vi "Query Status Register.vi"(8 "error in (no error)":errorcluster, 11 "IF_XX in":refnum<class "IF_XX.lvclass">) -> (0 "error out":errorcluster, 3 "IF_XX out":refnum<class "IF_XX.lvclass">)   [LabVIEW 2019, in "IF_XX.lvlib" / "IF_XX.lvclass"]
doc: "The implementation must read status registers and push the status register values to private data for:\nOCP Flag, OVP Flag, Interlock Flag, Output Flag into the private data arrays of the power supply class.\n\nThe routine queries the OVP and OCP registers, Although it is unclear what the return value is expected to be, so we'll have to determine during integration"
uses:
  Library/IF_XX.lvclass
  Library/IF_XX.lvclass/IF_XX.ctl
panel:
  out "Read data 3":string
  out "Read data 2":string
  out "Read data":string
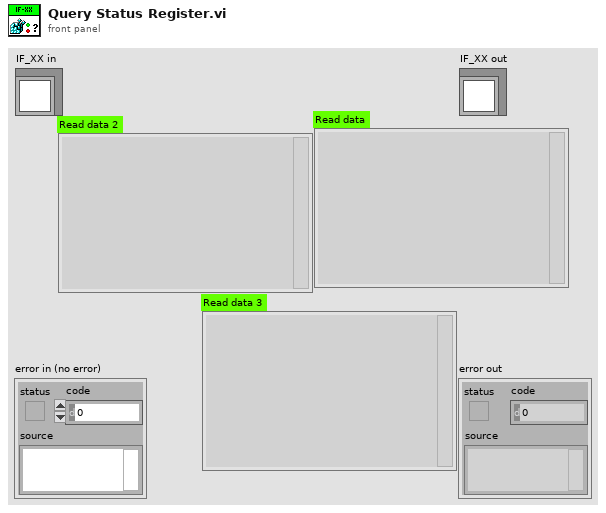
[diagram p1: front panel]
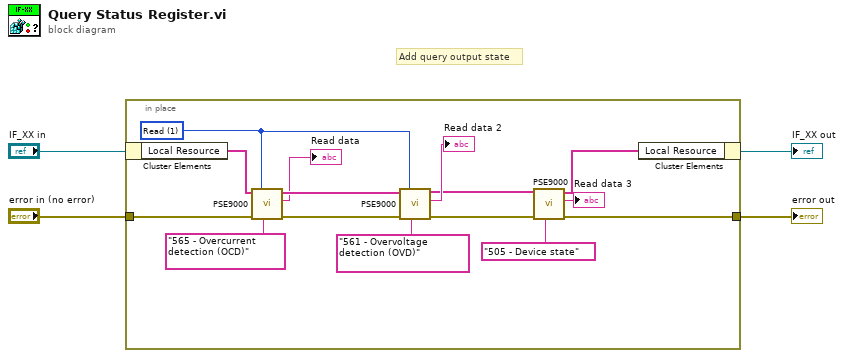
[diagram p0: block diagram]
diagram:
  # "Add query output state"
  n1 = in-place {
    in-place-border: "error in (no error)" -> [w16]
    in-place-border: [w7] -> w1
    w17 = u8 1 items=["Write", "Read"] ("Access")
    n2 = in-place-cluster #1("IF_XX in") -> ("Local Resource"=w18:string[])
    n3 = call <instrlib>:"PSE9000.vi"("Command list"="565 - Overcurrent detection (OCD)", "Error in"=w16, "Access"=w17, "Device information in"=w18) -> ("Error out"=w15:errorcluster, "Read data"=→"Read data":string, "Device information out"=w19:string[])  [unwired: 2 in, 1 out]
    n4 = call <instrlib>:"PSE9000.vi"("Command list"="561 - Overvoltage detection (OVD)", "Error in"=w15, "Access"=w17, "Device information in"=w19) -> ("Error out"=w8:errorcluster, "Read data"=→"Read data 2":string, "Device information out"=w10:string[])  [unwired: 2 in, 1 out]
    n5 = call <instrlib>:"PSE9000.vi"("Command list"="505 - Device state", "Error in"=w8, "Device information in"=w10) -> ("Error out"=w7:errorcluster, "Read data"=→"Read data 3":string, "Device information out"=w9:string[])  [unwired: 3 in, 1 out]
    n6 = in-place-cluster #1("Local Resource"=w9) -> (→"IF_XX out":refnum<class "IF_XX.lvclass">)
  }
  "error out" <- w1
